vi "Single Acquisition and RMS (Amplitude Reg) Test UI.vi"() -> ()   [LabVIEW 2014]
uses:
  <vilib>/FPGAPlugInAG/sbRIO-9636/niLvFpga_Open_sbRIO-9636.vi
  <vilib>/rvi/interface/common/dynamic/niFpgaDynamicAddResources.vi
  <vilib>/rvi/interface/common/niFpgaWaitOnOcc.vi
  <vilib>/Utility/error.llb/Error Cluster From Error Code.vi
  <vilib>/rvi/errors/niLvFpgaAdjustHostInterfaceError.vi
  <vilib>/FPGAPlugInAG/Dynamic/niLvFpga_Run_Dynamic.vi
  <vilib>/FPGAPlugInAG/Dynamic/niLvFpga_Close_Dynamic.vi
  <vilib>/rvi/interface/nirviOpenFPGA/nirviOpenFPGA.xnode
  FPGA Bitfiles/LaserDistanceSen_FPGATarget_RMSMeasurement(A_I9w0Pif+rIo.lvbitx
  FPGA Target/Test VIs/RMS Measurement (Amplitude Reg) Test.vi
  <vilib>/rvi/interface/nirviMethod/nirviMethod.xnode
  <vilib>/rvi/interface/nirviReadWriteControl/nirviReadWriteControl.xnode
  <vilib>/rvi/interface/nirviCloseFPGA/nirviCloseFPGA.xnode
  <vilib>/rvi/errors/niLvFpgaMergeErrorWithErrorCode.vi
  <vilib>/rvi/interface/Simulation/niFpgaSimulationCallBeginRW.vi
  <vilib>/FPGAPlugInAG/Dynamic/niLvFpga_ConfigureFifo_Dynamic.vi
  <vilib>/FPGAPlugInAG/Dynamic/niLvFpga_StartFifo_Dynamic.vi
  <vilib>/FPGAPlugInAG/Dynamic/niLvFpga_ReadFifo_Dynamic.vi
  NiFpgaLv.dll
panel:
  out "DC (Mean)":fxp<+/-,12,12>
  out "RMS":fxp<+,12,12>
  in  "Amplitude (0:1)":fxp<+,4,1>=1.0
  in  "Number of Elements to read":u32=2047
  out "Waveform Graph (input data)":dbl[](graph)
  out "Elements Remaining":u32
  # "Attenuazione: 0,69 (Gain)"
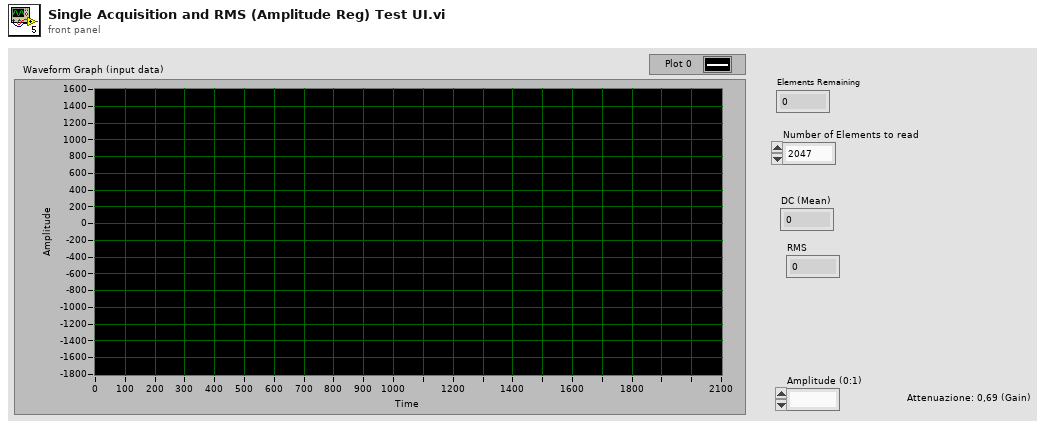
[diagram p1: front panel]
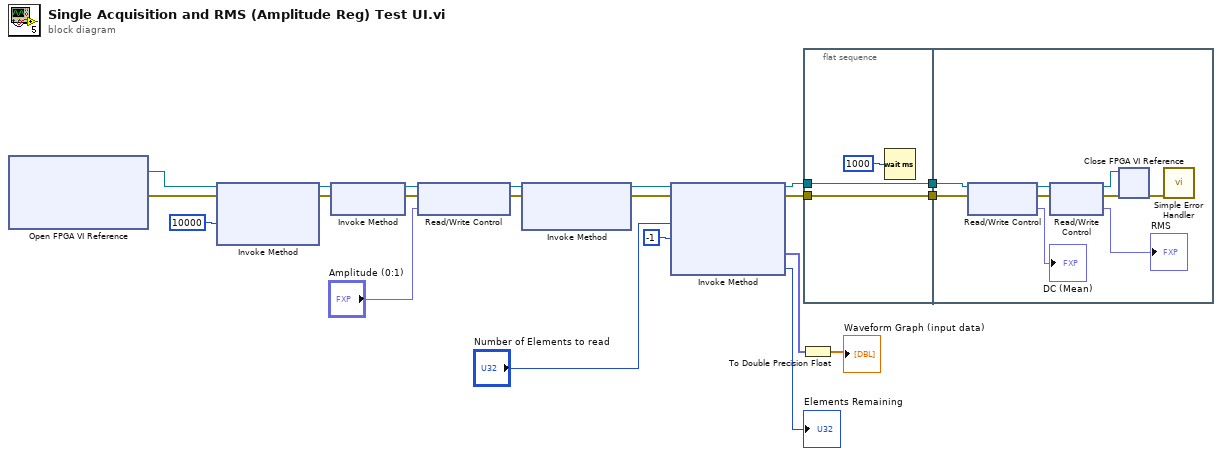
[diagram p0: block diagram]
diagram:
  n1 = xnode "Open FPGA VI Reference"() -> ("FPGA VI Reference Out"=w11:refnum<k20>, "error out"=w12:errorcluster)  [unwired: 2 in]
  n2 = xnode "Invoke Method"("FPGA VI Reference In"=w11, "error in"=w12, "Requested Depth"=u32 10000) -> ("FPGA VI Reference Out"=w19:refnum<k20>, "error out"=w20:errorcluster)  [unwired: 1 out]
  n3 = xnode "Invoke Method"("FPGA VI Reference In"=w19, "error in"=w20) -> ("FPGA VI Reference Out"=w10:refnum<k20>, "error out"=w9:errorcluster)
  n4 = xnode "Read/Write Control"("FPGA VI Reference In"=w10, "error in"=w9, "Amplitude (0:1)"="Amplitude (0:1)") -> ("FPGA VI Reference Out"=w7:refnum<k20>, "error out"=w8:errorcluster)
  n5 = xnode "Invoke Method"("FPGA VI Reference In"=w7, "error in"=w8) -> ("FPGA VI Reference Out"=w18:refnum<k20>, "error out"=w17:errorcluster)  [unwired: 1 in]
  n6 = xnode "Invoke Method"("FPGA VI Reference In"=w18, "error in"=w17, "Number of Elements"="Number of Elements to read", "Timeout (ms)"=-1) -> ("FPGA VI Reference Out"=w3:refnum<k20>, "error out"=w2:errorcluster, "Data"=w1:fxp<+/-,12,12>[], "Elements Remaining"=→"Elements Remaining":u32)
  n7 = To Double Precision Float(number=w1) -> (double precision float=→"Waveform Graph (input data)":dbl[])
  n8 = flat-sequence {
    tunnel: w2 -> [w23]
    tunnel: w3 -> [w24]
    tunnel: [w24] -> w5
    tunnel: [w23] -> w4
    tunnel: w5 -> [w30]
    tunnel: w4 -> [w29]
    frame #0 {
      n9 = Wait (ms)(milliseconds to wait=u32 1000) -> ()  [unwired: 1 out]
    }
    frame #1 {
      n10 = xnode "Read/Write Control"("FPGA VI Reference In"=w30, "error in"=w29) -> ("FPGA VI Reference Out"=w27:refnum<k20>, "error out"=w28:errorcluster, "DC (Mean)"=→"DC (Mean)":fxp<+/-,12,12>)
      n11 = xnode "Read/Write Control"("FPGA VI Reference In"=w27, "error in"=w28) -> ("FPGA VI Reference Out"=w26:refnum<k20>, "error out"=w25:errorcluster, "RMS"=→"RMS":fxp<+,12,12>)
      n12 = xnode "Close FPGA VI Reference"("FPGA VI Reference In"=w26, "error in"=w25) -> ("error out"=w31:errorcluster)
      n13 = call <vilib>:"Simple Error Handler.vi"("error in (no error)"=w31) -> ()  [unwired: 4 in, 5 out]
    }
  }
